vi "Interface initialize.vi"(8 "error in":errorcluster, 11 "Serial Master in":refnum<class "Serial Interface.lvclass">) -> (0 "error out":errorcluster, 3 "Serial Master out":refnum<class "Serial Interface.lvclass">)   [LabVIEW 2021, in "Serial Interface.lvclass"]
doc: "This provides an interface for the master to open a connection to the slave."
uses:
  Serial Interface.lvclass
  Serial Interface.lvclass/Serial Interface.ctl
  Network Protocol/Serial Shared Components/Serial Shared Components.lvlib
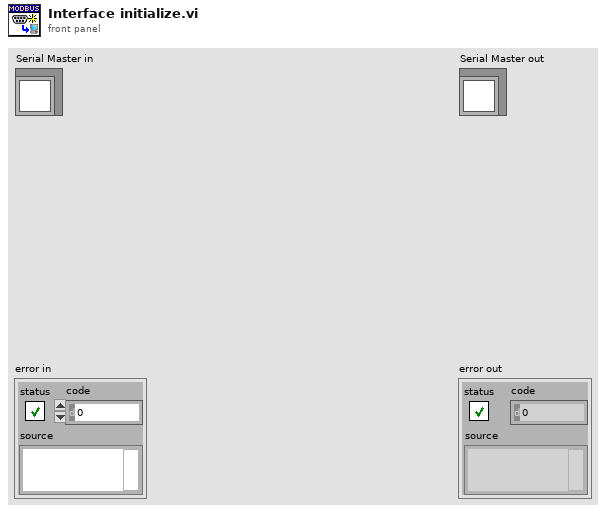
[diagram p1: front panel]
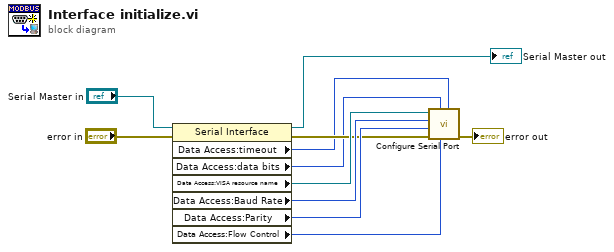
[diagram p0: block diagram]
diagram:
  n1 = property class="Serial Interface"(reference="Serial Master in", error in="error in") -> (reference out=→"Serial Master out":refnum<class "Serial Interface.lvclass">, error out=w3:errorcluster, "Data Access:timeout"=w2:u32, "Data Access:data bits"=w1:u16, "Data Access:VISA resource name"=w10:refnum<visa-resource-name>, "Data Access:Baud Rate"=w9:u32, "Data Access:Parity"=w8:u16, "Data Access:Flow Control"=w7:u16)
  n2 = call "Configure Serial Port.vi"("Timeout"=w2, "Flow Control"=w7, "data bits"=w1, "error in (no error)"=w3, "Parity"=w8, "Baud Rate"=w9, "VISA Refnum in"=w10) -> ("error out"=→"error out":errorcluster)  [unwired: 4 in]
